vi "Get Rack Number.vi"(8 "error in (no error)":errorcluster, 11 "S7NetCom in":refnum<class "S7NetCom.lvclass">) -> (0 "error out":errorcluster, 2 "Rack No.":u8 format="%0d", 3 "S7NetCom out":refnum<class "S7NetCom.lvclass">)   [LabVIEW 2014, in "S7NetCom.lvclass"]
doc: "____\nCopyright (c) 2019 Hampel Software Engineering (HSE), released under BSD license. More info can be found on https://dokuwiki.hampel-soft.com/code/hse/s7netcom. Original code published by Marc Christenson, Sisu Devices."
uses:
  S7NetCom.lvclass
  S7NetCom.lvclass/S7NetCom.ctl
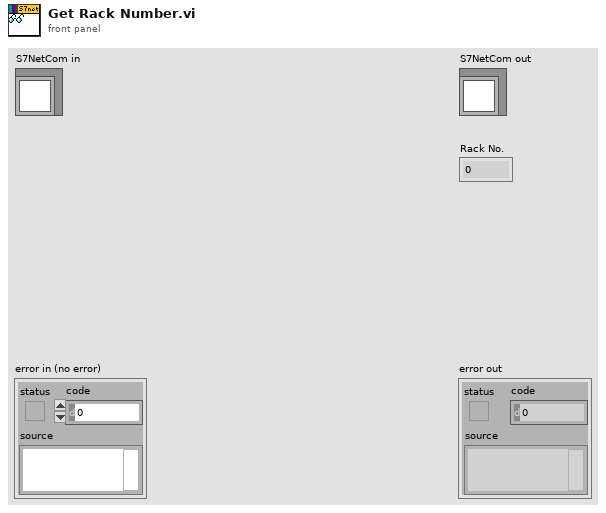
[diagram p1: front panel]
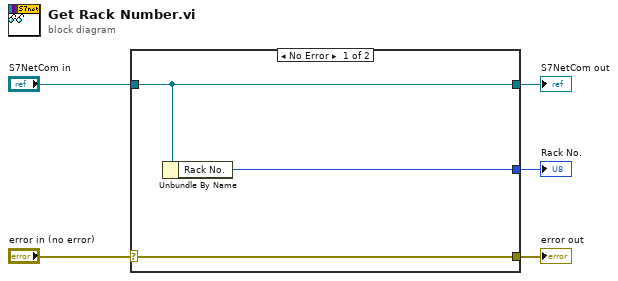
[diagram p0: block diagram]
diagram:
  n1 = case shown="No Error" "error in (no error)" {
    selector: "error in (no error)" -> [w8 w9]
    tunnel: [w8 w9] -> w4
    tunnel: [w7 w10] -> w2
    tunnel: "S7NetCom in" -> [w7 w10]
    tunnel: [w6 _] -> w1
    frame No Error {
      n2 = Unbundle By Name(w7) -> ("Rack No."=w6:u8)
    }
    frame Error {
    }
  }
  "error out" <- w4
  "S7NetCom out" <- w2
  "Rack No." <- w1
